vi "Deploy-Step-460-SynchronousInstallerUpload.vi"(0 "Deployment Engine":refnum<class "Deploy-DeploymentEngine.lvclass">, 11 "error in":errorcluster) -> (15 "error out":errorcluster)   [LabVIEW 2013]
uses:
  <resource>/Framework/Providers/Wirebird Labs LLC/Deploy/Support/Deployment Engine/Deploy-DeploymentEngine.lvclass
  <resource>/Framework/Providers/Wirebird Labs LLC/Deploy/Resources/Featherweight/Web/Transfer Client/Deploy-FTW-TransferClient.lvclass
panel:
  # "Inputs"
  # "Outputs"
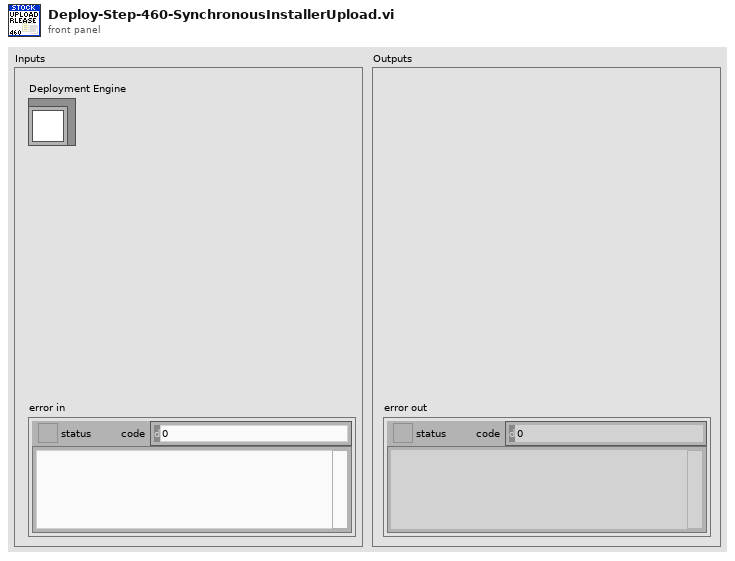
[diagram p1: front panel]
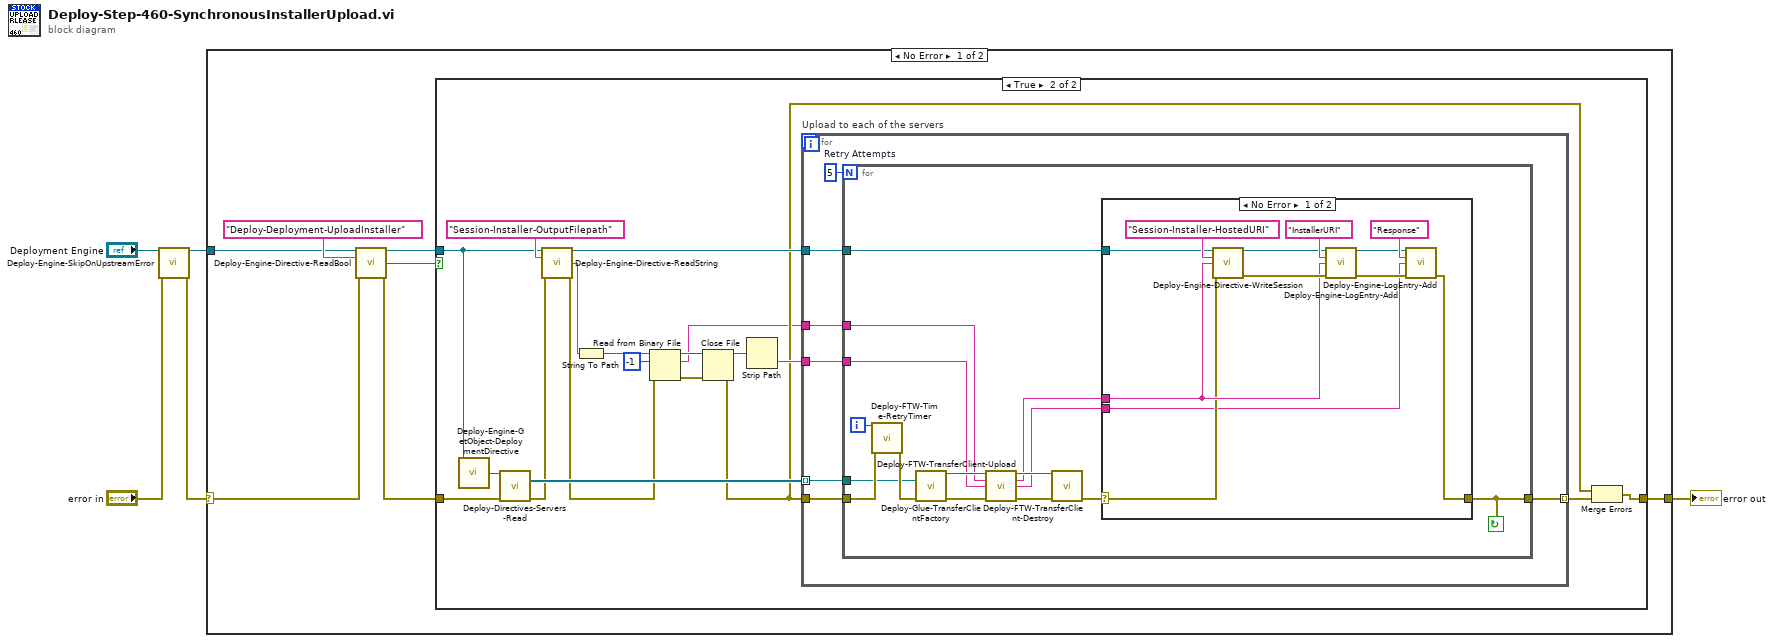
[diagram p0: block diagram]
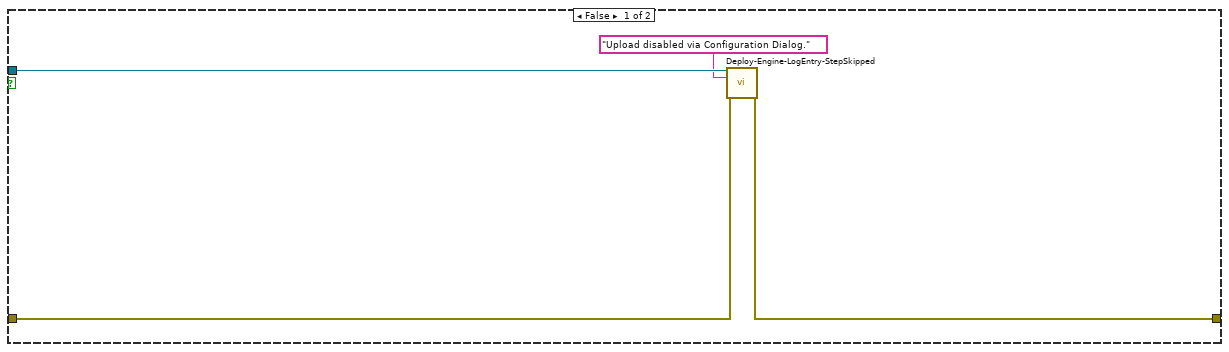
[diagram p2: hidden frame]
diagram:
  n1 = call <resource>:"Deploy-Engine-SkipOnUpstreamError.vi"("Engine"="Deployment Engine", "error in"="error in") -> ("Engine out"=w3:refnum<class "Deploy-DeploymentEngine.lvclass">, "error out"=w1:errorcluster)  [unwired: 12 in]
  n2 = case shown="No Error" w1 {
    selector: w1 -> [w8 w71]
    tunnel: [w12 w71] -> w5
    tunnel: w3 -> [w10 _]
    frame No Error {
      n3 = call <resource>:"Deploy-Engine-Directive-ReadBool.vi"("Engine"=w10, "Directive"="Deploy-Deployment-UploadInstaller" ("Property Name"), "error in"=w8) -> ("Engine out"=w9:refnum<class "Deploy-DeploymentEngine.lvclass">, "Value"=w6:bool, "error out"=w7:errorcluster)  [unwired: 10 in]
      n4 = case shown="True" w6 {
        tunnel: w9 -> [w16 w31]
        tunnel: w7 -> [w15 w34]
        tunnel: [w14 w27] -> w12
        frame False {
          n5 = call <resource>:"Deploy-Engine-LogEntry-StepSkipped.vi"("Engine"=w16, "Additional Information"="Upload disabled via Configuration Dialog.", "error in"=w15) -> ("error out"=w14:errorcluster)  [unwired: 11 in, 1 out]
        }
        frame True {
          n6 = call <resource>:"Deploy-Engine-GetObject-DeploymentDirective.vi"("Engine"=w31) -> ("Deployment Directives"=w35:refnum<class "Deploy-Directives.lvclass">)  [unwired: 3 in]
          n7 = call <resource>:"Deploy-Directives-Servers-Read.vi"("Deployment Directives"=w35, "error in"=w34) -> ("Deployment Servers"=w33:refnum<class "Deploy-DeploymentServer.lvclass">[], "error out"=w29:errorcluster)  [unwired: 10 in, 2 out]
          n8 = call <resource>:"Deploy-Engine-Directive-ReadString.vi"("Engine"=w31, "Directive"="Session-Installer-OutputFilepath", "error in"=w29) -> ("Engine out"=w30:refnum<class "Deploy-DeploymentEngine.lvclass">, "Resolved Value"=w26:string, "error out"=w19:errorcluster)  [unwired: 10 in]
          n9 = String To Path(string=w26) -> (path=w21:path)
          n10 = Read from Binary File(8:w19, 10:-1 ("count (1)"), 11:w21) -> (0:w22:errorcluster, 2:w17:string, 3:w23:refnum<file>)  [unwired: 3 in, 1 out]
          n11 = Close File(refnum=w23, error in=w22) -> (path=w20:path, error out=w18:errorcluster)
          n12 = Strip Path(path=w20) -> (name=w25:string)  [unwired: 1 out]
          n13 = for "Upload to each of the servers" {
            tunnel: [w42] -> w28 mode=indexing
            tunnel: w30 -> [w40]
            tunnel: w18 -> [w39]
            tunnel: w33 -> [w38] mode=indexing
            tunnel: w25 -> [w37]
            tunnel: w17 -> [w36]
            w41 = 5  # Retry Attempts
            n14 = for {
              N: w41 -> [_]
              tunnel: [w46] -> w42
              tunnel: w40 -> [w53]
              tunnel: w39 -> [w56]
              tunnel: w38 -> [w54]
              tunnel: w37 -> [w48]
              tunnel: w36 -> [w44]
              i -> [w57]
              stop <- w46 continue-if-true
              n15 = call <resource>:"Deploy-FTW-Time-RetryTimer.vi"("Retry Attempt (zero-indexed)"=w57, "error in"=w56) -> ("error out"=w55:errorcluster)  [unwired: 11 in, 2 out]
              n16 = call <resource>:"Deploy-Glue-TransferClientFactory.vi"("Deployment Server"=w54, "error in"=w55) -> ("Transfer Client"=w52:refnum<class "Deploy-FTW-TransferClient.lvclass">, "error out"=w50:errorcluster)  [unwired: 10 in, 2 out]
              n17 = call-dynamic "Deploy-FTW-TransferClient-Upload.vi"("Transfer Client"=w52, "Data"=w44, "Remote Filename"=w48, "error in"=w50) -> ("Transfer Client out"=w51:refnum<class "Deploy-FTW-TransferClient.lvclass">, "URI"=w47:string, "Response"=w43:string, "error out"=w49:errorcluster)  [unwired: 7 in, 1 out]
              n18 = call-dynamic "Deploy-FTW-TransferClient-Destroy.vi"("Transfer Client"=w51, "error in"=w49) -> ("error out"=w45:errorcluster)  [unwired: 13 in]
              n19 = case shown="No Error" w45 {
                selector: w45 -> [w63 w70]
                tunnel: w53 -> [w67 _]
                tunnel: w47 -> [w64 _]
                tunnel: [w59 w70] -> w46
                tunnel: w43 -> [w58 _]
                frame No Error {
                  n20 = call <resource>:"Deploy-Engine-Directive-WriteSession.vi"("Engine"=w67, "Directive"="Session-Installer-HostedURI", "Value"=w64, "error in"=w63) -> ("Engine out"=w66:refnum<class "Deploy-DeploymentEngine.lvclass">, "error out"=w65:errorcluster)  [unwired: 10 in]
                  n21 = call <resource>:"Deploy-Engine-LogEntry-Add.vi"("Engine"=w66, "Event Type"="InstallerURI", "Event Data"=w64, "error in"=w65) -> ("Engine out"=w60:refnum<class "Deploy-DeploymentEngine.lvclass">, "error out"=w61:errorcluster)  [unwired: 10 in]
                  n22 = call <resource>:"Deploy-Engine-LogEntry-Add.vi"("Engine"=w60, "Event Type"="Response", "Event Data"=w58, "error in"=w61) -> ("error out"=w59:errorcluster)  [unwired: 10 in, 1 out]
                }
                frame Error {
                }
              }
            }
          }
          n23 = Merge Errors(w18, w28) -> (w27:errorcluster)
        }
      }
    }
    frame Error {
    }
  }
  "error out" <- w5
